vi "Unflatten Names (String).vi"(0 "names in":string, 11 "error in (no error)":errorcluster) -> (4 "names out":string[](array[string]), 15 "error out":errorcluster)   [LabVIEW 2020, in "SLSC.lvlib"]
doc: "Converts a comma-delimited list of strings into an array of strings. If the list contains colon-delimited ranges, they will be expanded."
uses:
  <vilib>/SLSC/SLSC.lvlib
  nislsclvapi.dll
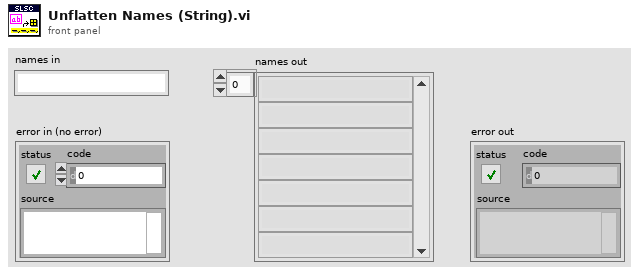
[diagram p1: front panel]
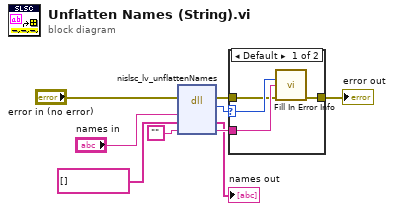
[diagram p0: block diagram]
diagram:
  n1 = dll-call lib="nislsclvapi.*" fn="nislsc_lv_unflattenNames"(error in="error in (no error)", "namesIn"="names in", "namesOut"=string[] [] ("contexts out"), "extendedErrorInfo"="") -> (error out=w7:errorcluster, "return type"=w6:i32, "namesOut"=→"names out":string[], "extendedErrorInfo"=w8:string)  [unwired: 3 in, 1 out]
  n2 = case shown="Default" w6 {
    selector: w6 -> [w13 _]
    tunnel: w8 -> [w12 _]
    tunnel: w7 -> [w11 w14]
    tunnel: [w10 w14] -> w1
    frame Default {
      n3 = call <vilib>:"Fill In Error Info.vi"("status code"=w13, "extended error info"=w12, "error in"=w11) -> ("error out"=w10:errorcluster)  [unwired: 12 in]
    }
    frame 0 {
    }
  }
  "error out" <- w1
